vi "GUI.Button.SetDisabled.vi"(7 "referenceToControls in":refnum<vi>[](array[refnum]), 8 "error in (no error)":errorcluster, 10 "buttonDisabled":T1(ring), 11 "buttonName":string) -> (0 "error out":errorcluster, 5 "referenceToControls out":refnum<vi>[](array[refnum]))   [LabVIEW 2019]
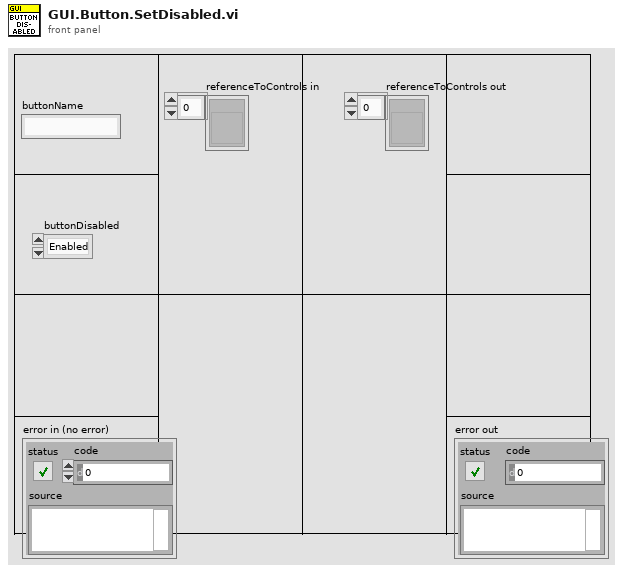
[diagram p1: front panel]
types:
  T1 = enum8{"Enabled", "Disabled", "Disabled and Grayed Out"}
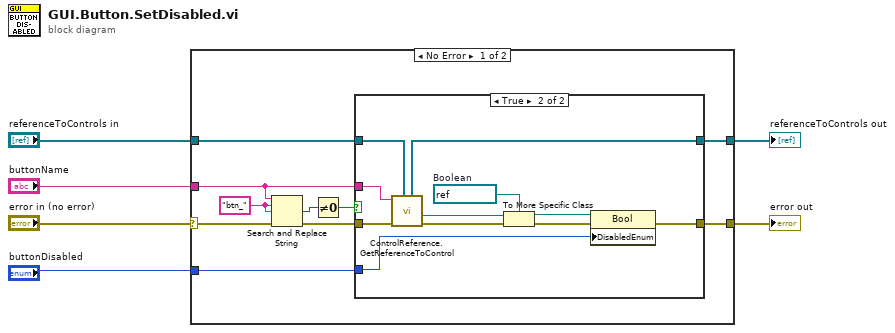
[diagram p0: block diagram]
diagram:
  n1 = case shown="No Error" "error in (no error)" {
    selector: "error in (no error)" -> [w14 w31]
    tunnel: [w16 w31] -> w4
    tunnel: "buttonName" -> [w12 _]
    tunnel: "referenceToControls in" -> [w9 w30]
    tunnel: [w8 w30] -> w6
    tunnel: "buttonDisabled" -> [w7 _]
    frame No Error {
      w15 = "btn_"
      n2 = Search and Replace String(input string=w12, search string=w15, replace string=w15, error in=w14) -> (number of replacements=w11:i32, error out=w13:errorcluster)  [unwired: 4 in, 2 out]
      n3 = Not Equal To 0?(x=w11) -> (x != 0?=w10:bool)
      n4 = case shown="True" w10 {
        tunnel: w13 -> [w18 w24]
        tunnel: w9 -> [w17 w23]
        tunnel: w12 -> [_ w22]
        tunnel: [w18 w25] -> w16
        tunnel: [w17 w20] -> w8
        tunnel: w7 -> [_ w19]
        frame False {
        }
        frame True {
          w28 = refnum<vi> refnum  # Boolean
          n5 = call "ControlReference.GetReferenceToControl.vi"("referenceToControls in"=w23, "error in (no error)"=w24, "controlLabelText"=w22) -> ("error out"=w26:errorcluster, "referenceToControl"=w21:refnum<vi>, "referenceToControls out"=w20:refnum<vi>[])  [unwired: 6 in]
          n6 = To More Specific Class(target class=w28, reference=w21, error in=w26) -> (specific class reference=w27:refnum<vi>, error out=w29:errorcluster)
          n7 = property class="Bool"(reference=w27, error in=w29, "DisabledEnum"=w19) -> (error out=w25:errorcluster)  [unwired: 1 out]
        }
      }
    }
    frame Error {
    }
  }
  "referenceToControls out" <- w6
  "error out" <- w4
